vi "UnreserveSessions.vi"(6 "Session manager service gRPC ID":T4, 7 "Discovery service gRPC ID":T4, 8 "error in":errorcluster, 11 "sessions":T1[](array[typedef])) -> (0 "error out":errorcluster)   [LabVIEW 2020]
uses:
  <vilib>/gRPC/LabVIEW gRPC Library/Shared/grpcId.ctl
  <vilib>/MeasurementLink/MeasurementLink Session Management Client/RPC Messages/ni_measurementlink_sessionmanagement_v1_SessionInformation.ctl
  <vilib>/MeasurementLink/MeasurementLink Session Management Client/RPC Messages/nidevice_grpc_Session.ctl
  <vilib>/MeasurementLink/MeasurementLink Session Management Client/RPC Messages/ni_measurementlink_sessionmanagement_v1_ChannelMapping.ctl
  <vilib>/MeasurementLink/MeasurementLink Session Management Client/RPC Messages/ni_measurementlink_sessionmanagement_v1_UnreserveSessionsRequest.ctl
  <vilib>/MeasurementLink/MeasurementLink Discovery Client/MeasurementLink Discovery Client.lvlib
  <vilib>/MeasurementLink/MeasurementLink Session Management Client/MeasurementLink Session Management Client.lvlib
  <vilib>/gRPC/LabVIEW gRPC Library/grpc-lvsupport-release.lvlib
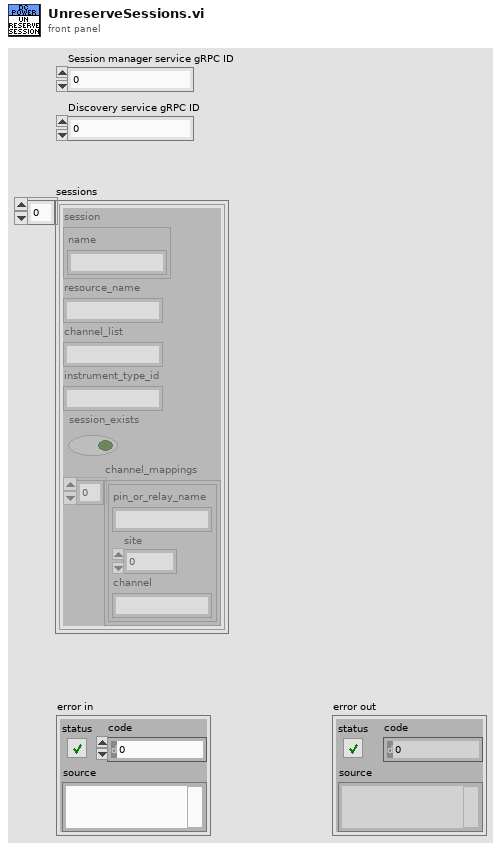
[diagram p1: front panel]
types:
  T1 = typedef "MeasurementLink Session Management Client.lvlib/ni_measurementlink_sessionmanagement_v1_SessionInformation.ctl" = cluster{"session":T2, "resource_name":string, "channel_list":string, "instrument_type_id":string, "session_exists":bool, "channel_mappings":T3[]}
  T2 = typedef "MeasurementLink Session Management Client.lvlib/nidevice_grpc_Session.ctl" = cluster{"name":string}
  T3 = typedef "MeasurementLink Session Management Client.lvlib/ni_measurementlink_sessionmanagement_v1_ChannelMapping.ctl" = cluster{"pin_or_relay_name":string, "site":i32, "channel":string}
  T4 = typedef "grpc-lvsupport-release.lvlib/grpcId.ctl" = u64
  T5 = typedef "MeasurementLink Session Management Client.lvlib/ni_measurementlink_sessionmanagement_v1_UnreserveSessionsRequest.ctl" = cluster{"sessions":T1[]}
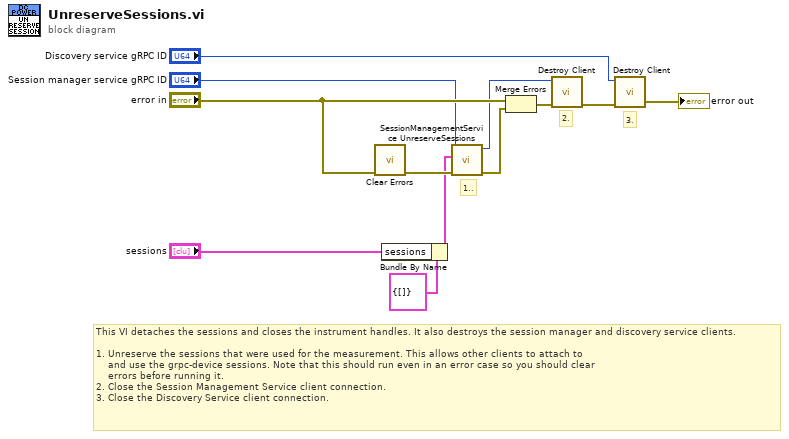
[diagram p0: block diagram]
diagram:
  # "This VI detaches the sessions and closes the instrument handles. It also destroys the session manager and discovery service clients.\n\n1. Unreserve the sessions that were used for the measurement. This allows other clients to attach to\n    and use the grpc-device sessions. Note that this should run even in an error case so you should clear \n    errors before running it.\n2. Close the Session Management Service client connection.\n3. Close the Discovery Service client connection."
  # "1.."
  # "3."
  # "2."
  n1 = call <vilib>:"Clear Errors.vi"("error in (no error)"="error in") -> ("error out"=w9:errorcluster)  [unwired: 5 in, 1 out]
  n2 = Bundle By Name(cluster=T5 {"sessions"=[]} ("Request Data"), "sessions"="sessions") -> (w7:T5)
  n3 = call <vilib>:"SessionManagementService UnreserveSessions.vi"("error in"=w9, "Request Data"=w7, "gRPC ID"="Session manager service gRPC ID") -> ("error out"=w5:errorcluster, "gRPC ID out"=w11:T4)  [unwired: 6 in, 1 out]
  n4 = Merge Errors("error in", w5) -> (w6:errorcluster)
  n5 = call <vilib>:"Destroy Client.vi"("error in"=w6, "gRPC ID"=w11) -> ("error out"=w10:errorcluster)  [unwired: 9 in]
  n6 = call <vilib>:"Destroy Client.vi"("error in"=w10, "gRPC ID"="Discovery service gRPC ID") -> ("error out"=→"error out":errorcluster)  [unwired: 9 in]
